vi "Execute Query.vi"(8 "error in (no error)":errorcluster, 10 "SQL query":string, 11 "MYSQL Database in":refnum<class "MYSQL Server.lvclass">) -> (0 "error out":errorcluster, 3 "MYSQL Database out":refnum<class "MYSQL Server.lvclass">)   [LabVIEW 2023, in "HardwareAbstractionLayer_LVOOP.lvlib" / "MYSQL Server.lvclass"]
uses:
  MYSQL Server.lvclass
  MYSQL Server.lvclass/MYSQL Server.ctl
  <vilib>/addons/database/Connection.llb/Conn Execute.vi
  <vilib>/addons/database/Recordset.llb/Rec Destroy - Connection.vi
  <vilib>/addons/database/NI_Database_API.lvlib
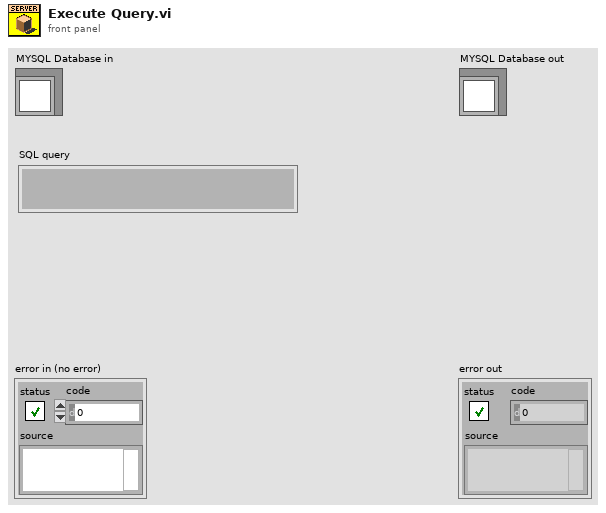
[diagram p1: front panel]
types:
  T1 = typedef "NI_Database_API.lvlib/Conn ObjectReference.ctl" = refnum<k1>
  T2 = typedef "NI_Database_API.lvlib/Rec ObjectReference.ctl" = refnum<k1>
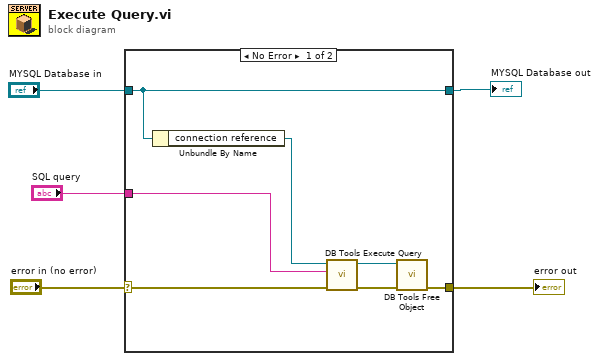
[diagram p0: block diagram]
diagram:
  n1 = case shown="No Error" "error in (no error)" {
    selector: "error in (no error)" -> [w9 w14]
    tunnel: "MYSQL Database in" -> [w12 w13]
    tunnel: [w7 w14] -> w3
    tunnel: [w12 w13] -> w2
    tunnel: "SQL query" -> [w10 _]
    frame No Error {
      n2 = Unbundle By Name(w12) -> ("connection reference"=w11:T1)
      n3 = call-poly <vilib>:"DB Tools Execute Query.vi"("error in (no error)"=w9, "SQL query"=w10, "connection reference"=w11) -> ("error out"=w8:errorcluster, "recordset reference"=w6:T2)  [unwired: 5 in]
      n4 = call-poly <vilib>:"DB Tools Free Object.vi"("error in (no error)"=w8, "recordset reference"=w6) -> ("error out"=w7:errorcluster)  [unwired: 8 in, 1 out]
    }
    frame Error {
    }
  }
  "error out" <- w3
  "MYSQL Database out" <- w2
